vi "Parse-attribute.vi"(8 "error in (no error)":errorcluster, 10 "String in":string, 11 "EnableLaser in":refnum<class "EnableLaser.lvclass">) -> (0 "error out":errorcluster, 1 "Valid attribute?":bool, 2 "Remaining string":string, 3 "EnableLaser out":refnum<class "EnableLaser.lvclass">)   [LabVIEW 2013, in "HardwareCharacterization.lvlib" / "EnableLaser.lvclass"]
uses:
  EnableLaser.lvclass
  Attributes.ctl
  Attribute-ID.ctl
  Attribute-XML.lvclass/Attribute-XML.ctl
  ID.lvclass/ID.ctl
  Boolean/Boolean.lvclass/Boolean.ctl
  Write Attribute.vi
  Write ID-attribute.vi
  Boolean/Write Boolean.vi
  Attribute-XML.lvclass
  ID.lvclass
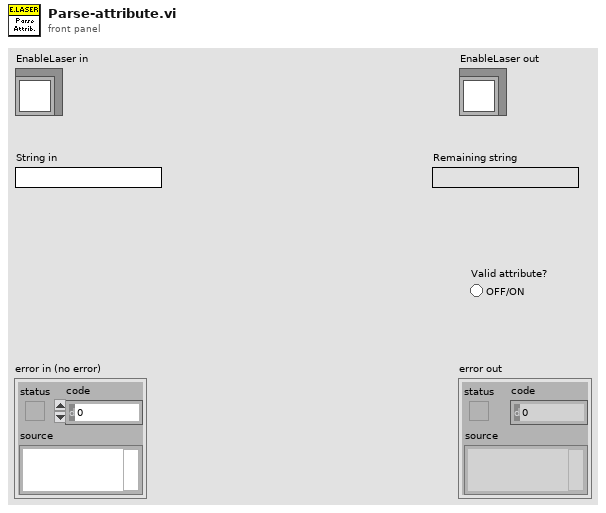
[diagram p1: front panel]
types:
  T1 = typedef "HardwareCharacterization.lvlib/ID.lvclass/Attribute-ID.ctl" = enum16{"FieldOffset", "TransformEnable", "Transform", "Units", "XYCalFactor", "EnableLaser", "JumpDelay", "MarkDelay", "PolyDelay", "LaserOnDelay", "LaserOffDelay", "JumpSpeed", "MarkSpeed", "LaserPowerDelay", "LaserEnableDelay", "LaserPower", "Offset"}
  T2 = typedef "HardwareCharacterization.lvlib/Attribute-XML.lvclass/Attributes.ctl" = enum16{"id"}
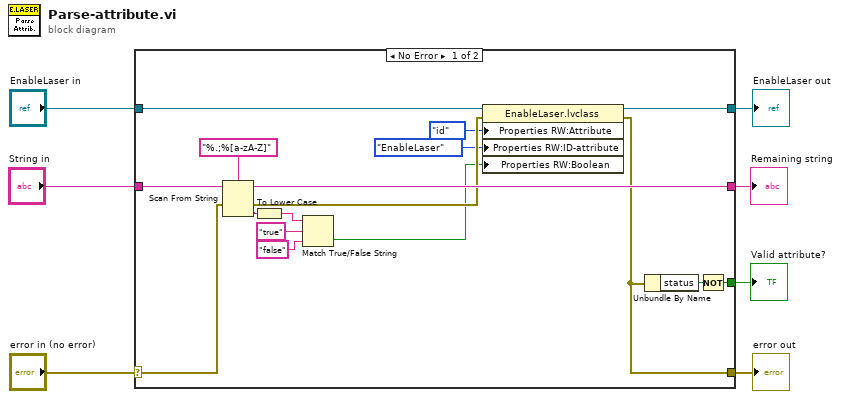
[diagram p0: block diagram]
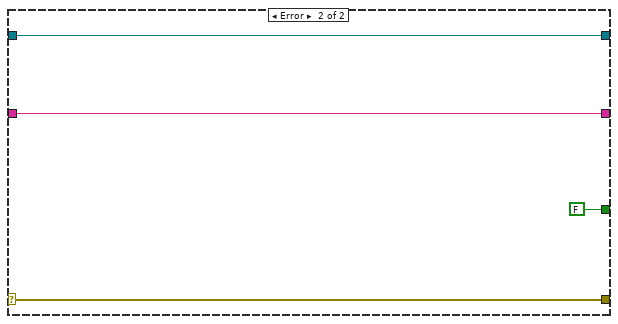
[diagram p2: hidden frame]
diagram:
  n1 = case shown="No Error" "error in (no error)" {
    selector: "error in (no error)" -> [w21 w28]
    tunnel: [w11 w28] -> w6
    tunnel: [w18 w27] -> w4
    tunnel: "EnableLaser in" -> [w19 w27]
    tunnel: "String in" -> [w22 w26]
    tunnel: [w20 w26] -> w2
    tunnel: [w12 FALSE] -> w1
    frame No Error {
      n2 = Scan From String(format string="%.;%[a-zA-Z]", input string=w22, error in=w21) -> (remaining string=w20:string, error out=w17:errorcluster, output 1=w16:string)  [unwired: 2 in, 1 out]
      n3 = To Lower Case(string=w16) -> (all lower case string=w13:string)
      n4 = Match True/False String(2:"false" ("false string"), 3:"true" ("true string"), 4:w13) -> (0:w10:bool)  [unwired: 1 out]
      n5 = property class="EnableLaser.lvclass"(reference=w19, error in=w17, "Properties RW:Attribute"=Attributes."id" ("Attribute"), "Properties RW:ID-attribute"=Attribute-ID."EnableLaser" ("ID-attribute"), "Properties RW:Boolean"=w10) -> (reference out=w18:refnum<class "EnableLaser.lvclass">, error out=w11:errorcluster)
      n6 = Unbundle By Name(w11) -> ("status"=w23:bool)
      n7 = Not(x=w23) -> (.not. x?=w12:bool)
    }
    frame Error {
    }
  }
  "error out" <- w6
  "EnableLaser out" <- w4
  "Remaining string" <- w2
  "Valid attribute?" <- w1
